vi "IMAQdx LL-Event.vi"(8 "ErrIn":errorcluster, 11 "Camera":refnum<k21> caption="IMAQdx Session") -> (0 "ErrOut":errorcluster, 3 "ImgOut":T1)   [LabVIEW 2013]
doc: "Use this template to build a VI to use as a subVI."
uses:
  <vilib>/vision/Image Controls.llb/IMAQ Image.ctl
  <vilib>/vision/driver/IMAQdx.llb/IMAQdx Acquisition Mode.ctl
  <vilib>/vision/driver/IMAQdx.llb/IMAQdx Buffer Number Mode.ctl
  <vilib>/vision/driver/NI_Vision_Acquisition_Software.lvlib
  <resource>/objmgr/imaqdx.rc
panel:
  in  "stop":bool
  out "Frame Rate":dbl
  # "Input Parameters"
  # "Output Parameters"
  # "VI Description:\nThis VI is created to snap a image from imaging device."
  # ":: MVI Framework V1.0 ::\nAuthor:Gaoke Yang\nEmail: gaoke.yang@yahoo.com\nWeb: www.mvicontrol.com\nCopyright (C) 2013, MVI Technologies All Rights Reserved"
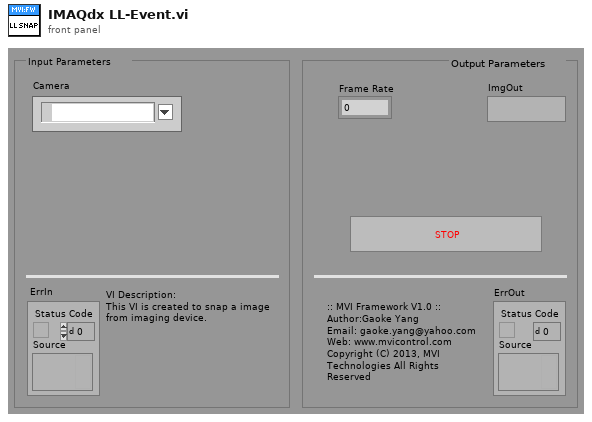
[diagram p1: front panel]
types:
  T1 = typedef "IMAQ Image.ctl" = refnum<image>
  T2 = typedef "NI_Vision_Acquisition_Software.lvlib/IMAQdx Acquisition Mode.ctl" = enum32{"One Shot", "Continuous"}
  T3 = typedef "IMAQdx.ctl" = refnum<k21>
  T4 = typedef "NI_Vision_Acquisition_Software.lvlib/IMAQdx Buffer Number Mode.ctl" = enum32{"Next", "Last", "Buffer Number"}
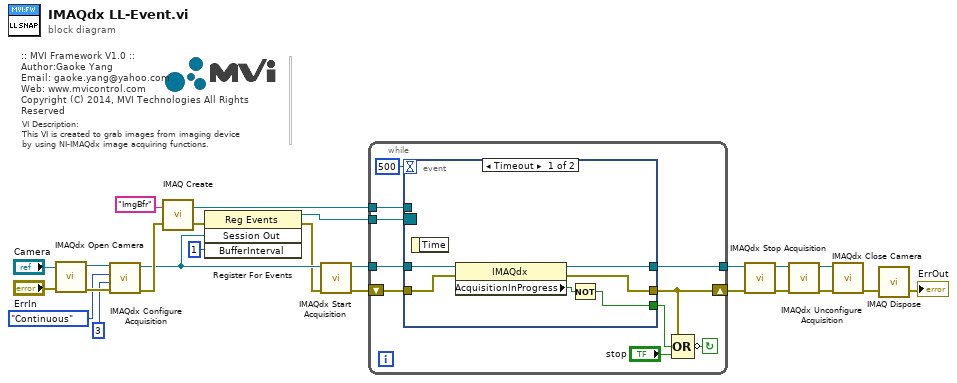
[diagram p0: block diagram]
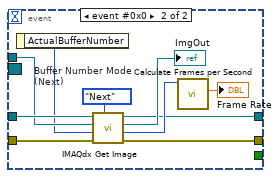
[diagram p2: hidden frame]
diagram:
  # "VI Description:\nThis VI is created to grab images from imaging device \nby using NI-IMAQdx image acquiring functions."
  # ":: MVI Framework V1.0 ::\nAuthor:Gaoke Yang\nEmail: gaoke.yang@yahoo.com\nWeb: www.mvicontrol.com\nCopyright (C) 2014, MVI Technologies All Rights Reserved"
  n1 = call <vilib>:"IMAQdx Open Camera.vi"("error in"="ErrIn", "Session In"="Camera") -> ("error out"=w19:errorcluster, "Session Out"=w20:T3)  [unwired: 8 in]
  n2 = call <vilib>:"IMAQdx Configure Acquisition.vi"("error in"=w19, "Number of Buffers"=u32 3, "Continuous?"=IMAQdx_Acquisition_Mode."Continuous", "Session In"=w20) -> ("error out"=w16:errorcluster, "Session Out"=w4:T3)  [unwired: 6 in]
  n3 = call "IMAQ Create"("Image Name"="ImgBfr" ("ImgBfr"), "error in (no error)"=w16) -> ("New Image"=w13:T1, "error out"=w5:errorcluster)  [unwired: 2 in, 1 out]
  n4 = register-events(error in=w5, w4, u32 1 ("BufferInterval")) -> (reference out=w1:refnum<event-registration>, error out=w2:errorcluster)  [unwired: 1 in]
  n5 = call <vilib>:"IMAQdx Start Acquisition.vi"("error in"=w2, "Session In"=w4) -> ("error out"=w14:errorcluster, "Session Out"=w15:T3)  [unwired: 8 in]
  n6 = while {
    shift-left: w14 -> [w31]
    shift-right: [w27] -> w10
    tunnel: w15 -> [w32]
    tunnel: w13 -> [w30]
    tunnel: [w29] -> w9
    tunnel: w1 -> [w28]
    stop <- w33 continue-if-true
    n7 = event shown="[0] Timeout" {
      selector: w28 -> [_ _]
      dyn-events: _ -> [_ _]
      timeout: 500 -> [_ _]
      tunnel: w32 -> [w40 w46]
      tunnel: w31 -> [w39 w45]
      tunnel: w30 -> [_ w42]
      tunnel: [w37 w43] -> w29
      tunnel: [w38 w44] -> w27
      tunnel: [w35 _] -> w25
      event Timeout {
        n8 = event-data() -> ()  [unwired: 1 in, 1 out]
        n9 = property class="IMAQdx"(reference=w40, error in=w39) -> (reference out=w37:T3, error out=w38:errorcluster, "AcquisitionInProgress"=w36:bool)
        n10 = Not(x=w36) -> (.not. x?=w35:bool)
      }
      event event #0x0 {
        w49 = IMAQdx_Buffer_Number_Mode."Next"  # Buffer Number Mode (Next)
        n11 = event-data() -> ("ActualBufferNumber"=w41:u32)  [unwired: 1 in]
        n12 = call <vilib>:"IMAQdx Get Image.vi"("Buffer Number Mode (Next)"=w49, "error in"=w45, "Buffer Number In"=w41, "Image In"=w42, "Session In"=w46) -> ("error out"=w44:errorcluster, "Buffer Number Out"=w47:u32, "Image Out"=→"ImgOut":T1, "Session Out"=w43:T3)  [unwired: 3 in]
        n13 = call <vilib>:"Calculate Frames per Second.vi"("Buffer Number"=w47) -> ("Processed Frames/s"=→"Frame Rate":dbl)  [unwired: 8 in, 2 out]
      }
    }
    n14 = Compound Arithmetic op=OR(w27, w25, "stop") -> (invert w33:bool)
  }
  n15 = call <vilib>:"IMAQdx Stop Acquisition.vi"("error in"=w10, "Session In"=w9) -> ("error out"=w8:errorcluster, "Session Out"=w23:T3)  [unwired: 8 out]
  n16 = call <vilib>:"IMAQdx Unconfigure Acquisition.vi"("error in"=w8, "Session In"=w23) -> ("error out"=w7:errorcluster, "Session Out"=w24:T3)  [unwired: 8 out]
  n17 = call <vilib>:"IMAQdx Close Camera.vi"("error in"=w7, "Session In"=w24) -> ("error out"=w6:errorcluster)  [unwired: 9 out]
  n18 = call "IMAQ Dispose"("error in (no error)"=w6) -> ("error out"=→"ErrOut":errorcluster)  [unwired: 2 in, 3 out]
